vi "SSC DCPower Configure Output Enabled And Connected V2.vi"(0 "DCPower SSC in":T1[](array[typedef]), 5 "Output Enabled And Connected":bool, 11 "error in":errorcluster) -> (4 "DCPower SSC out":T1[](array[typedef]), 15 "error out":errorcluster)   [LabVIEW 2019]
doc: "This VI configures output enabled and connected on the channels.\n\nT - Enable and then connect\nF - Disconnect and then disable"
uses:
  SSC DCPower.ctl
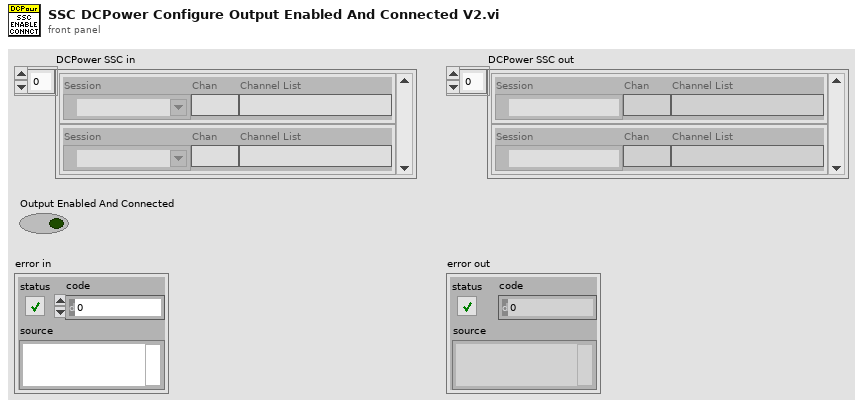
[diagram p1: front panel]
types:
  T1 = typedef "SSC DCPower.ctl" = cluster{"Session":refnum<k15>, "Chan":string, "Channel List":string}
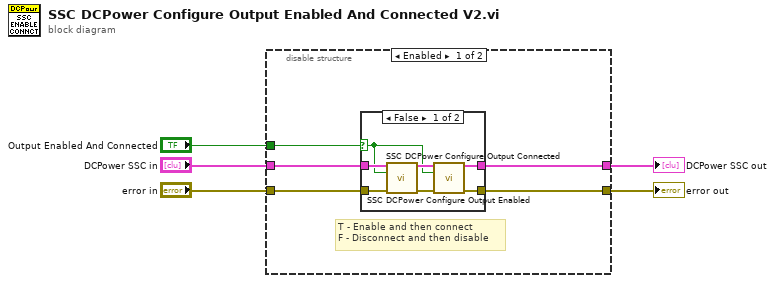
[diagram p0: block diagram]
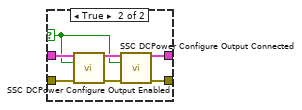
[diagram p2: hidden frame]
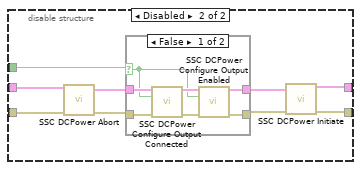
[diagram p3: hidden frame]
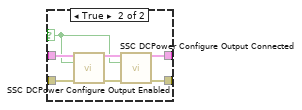
[diagram p4: hidden frame]
diagram:
  n1 = disable-structure shown="Enabled" {
    disable-tunnel: "error in" -> [w10 w33]
    disable-tunnel: [w9 w27] -> w4
    disable-tunnel: "DCPower SSC in" -> [w8 w31]
    disable-tunnel: [w7 w28] -> w2
    disable-tunnel: "Output Enabled And Connected" -> [w6 w25]
    frame Enabled {
      # "T - Enable and then connect\nF - Disconnect and then disable"
      n2 = case shown="False" w6 {
        selector: w6 -> [w11 w18]
        tunnel: w10 -> [w17 w24]
        tunnel: [w14 w21] -> w9
        tunnel: w8 -> [w15 w22]
        tunnel: [w12 w19] -> w7
        frame False {
          n3 = call "SSC DCPower Configure Output Connected.vi"("DCPower SSC in"=w15, "Output Connected"=w11, "error in"=w17) -> ("DCPower SSC out"=w13:T1[], "error out"=w16:errorcluster)  [unwired: 11 in]
          n4 = call "SSC DCPower Configure Output Enabled.vi"("DCPower SSC in"=w13, "Output Enabled"=w11, "error in"=w16) -> ("DCPower SSC out"=w12:T1[], "error out"=w14:errorcluster)  [unwired: 11 in]
        }
        frame True {
          n5 = call "SSC DCPower Configure Output Enabled.vi"("DCPower SSC in"=w22, "Output Enabled"=w18, "error in"=w24) -> ("DCPower SSC out"=w20:T1[], "error out"=w23:errorcluster)  [unwired: 11 in]
          n6 = call "SSC DCPower Configure Output Connected.vi"("DCPower SSC in"=w20, "Output Connected"=w18, "error in"=w23) -> ("DCPower SSC out"=w19:T1[], "error out"=w21:errorcluster)  [unwired: 11 in]
        }
      }
    }
    frame Disabled {
      n7 = call "SSC DCPower Abort.vi"("DCPower SSC in"=w31, "error in"=w33) -> ("DCPower SSC out"=w32:T1[], "error out"=w30:errorcluster)  [unwired: 12 in]
      n8 = case shown="False" w25 {
        selector: w25 -> [w34 w41]
        tunnel: w30 -> [w40 w47]
        tunnel: [w37 w44] -> w26
        tunnel: w32 -> [w38 w45]
        tunnel: [w35 w42] -> w29
        frame False {
          n9 = call "SSC DCPower Configure Output Connected.vi"("DCPower SSC in"=w38, "Output Connected"=w34, "error in"=w40) -> ("DCPower SSC out"=w36:T1[], "error out"=w39:errorcluster)  [unwired: 11 in]
          n10 = call "SSC DCPower Configure Output Enabled.vi"("DCPower SSC in"=w36, "Output Enabled"=w34, "error in"=w39) -> ("DCPower SSC out"=w35:T1[], "error out"=w37:errorcluster)  [unwired: 11 in]
        }
        frame True {
          n11 = call "SSC DCPower Configure Output Enabled.vi"("DCPower SSC in"=w45, "Output Enabled"=w41, "error in"=w47) -> ("DCPower SSC out"=w43:T1[], "error out"=w46:errorcluster)  [unwired: 11 in]
          n12 = call "SSC DCPower Configure Output Connected.vi"("DCPower SSC in"=w43, "Output Connected"=w41, "error in"=w46) -> ("DCPower SSC out"=w42:T1[], "error out"=w44:errorcluster)  [unwired: 11 in]
        }
      }
      n13 = call "SSC DCPower Initiate.vi"("DCPower SSC in"=w29, "error in"=w26) -> ("DCPower SSC out"=w28:T1[], "error out"=w27:errorcluster)  [unwired: 12 in]
    }
  }
  "error out" <- w4
  "DCPower SSC out" <- w2
